vi "WILT Find And Reserve Semaphore.vi"(8 "error in (no error)":errorcluster, 10 "Semaphore":T1[](array[typedef]), 11 "VISA Refnum in":refnum<visa-resource-name>) -> (0 "error out":errorcluster, 2 "Skip Semaphore":bool, 3 "Refnum out":T1)   [LabVIEW 2016]
uses:
  <vilib>/Utility/error.llb/whitespace.ctl
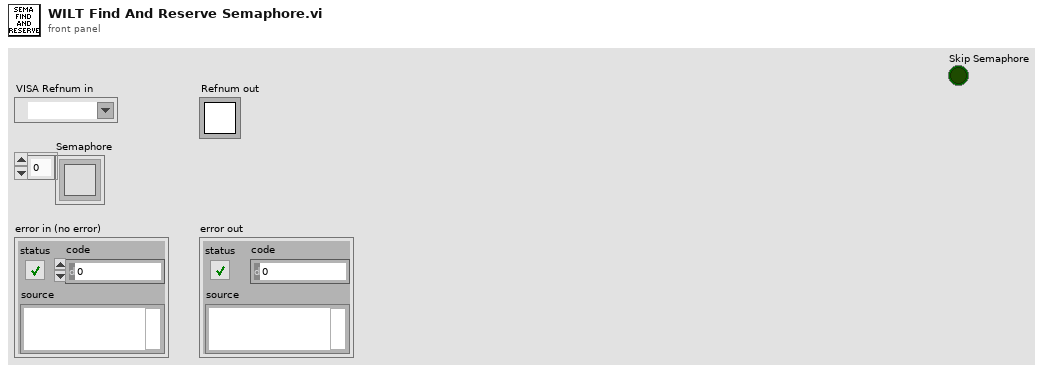
[diagram p1: front panel]
types:
  T1 = typedef "Semaphore RefNum" = refnum<k1>
  T2 = typedef "whitespace.ctl" = u16
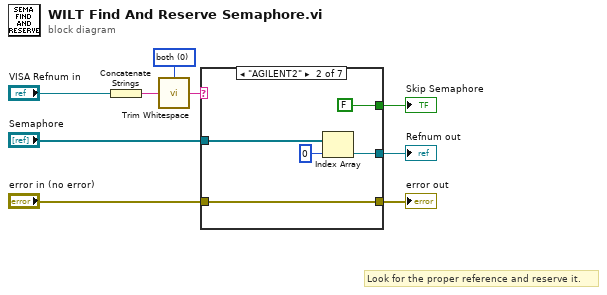
[diagram p0: block diagram]
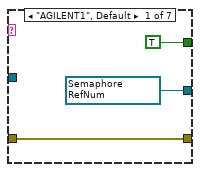
[diagram p2: hidden frame]
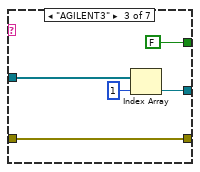
[diagram p3: hidden frame]
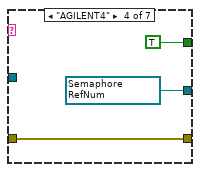
[diagram p4: hidden frame]
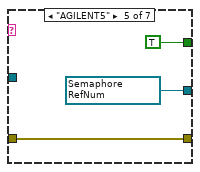
[diagram p5: hidden frame]
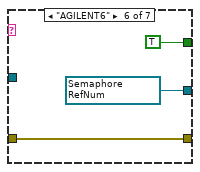
[diagram p6: hidden frame]
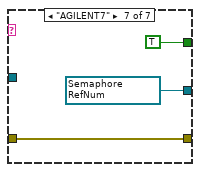
[diagram p7: hidden frame]
diagram:
  w5 = T2 0 items=["both", "start of string", "end of string"] ("location (both)")
  # "Look for the proper reference and reserve it."
  n1 = Concatenate Strings("VISA Refnum in") -> (w4:string)
  n2 = call <vilib>:"Trim Whitespace.vi"("string"=w4, "location (both)"=w5) -> ("trimmed string"=w6:string)
  n3 = case shown="\"AGILENT2\"" w6 {
    tunnel: "Semaphore" -> [_ w16 w21 _ _ _ _]
    tunnel: [w11 w15 w20 w24 w27 w30 w32] -> w7
    tunnel: [w12 w14 w19 w25 w28 w31 w34] -> w9
    tunnel: "error in (no error)" -> [w12 w14 w19 w25 w28 w31 w34]
    tunnel: [TRUE FALSE FALSE TRUE TRUE TRUE TRUE] -> w1
    frame "AGILENT1", Default {
      w11 = T1 refnum items=["semaphore"] ("Agilent")
    }
    frame "AGILENT2" {
      n4 = Index Array(array=w16, index=0) -> (element=w15:T1)
    }
    frame "AGILENT3" {
      n5 = Index Array(array=w21, index=1) -> (element=w20:T1)
    }
    frame "AGILENT4" {
      w24 = T1 refnum items=["semaphore"] ("Agilent")
    }
    frame "AGILENT5" {
      w27 = T1 refnum items=["semaphore"] ("Agilent")
    }
    frame "AGILENT6" {
      w30 = T1 refnum items=["semaphore"] ("Agilent")
    }
    frame "AGILENT7" {
      w32 = T1 refnum items=["semaphore"] ("Agilent")
    }
  }
  "error out" <- w9
  "Refnum out" <- w7
  "Skip Semaphore" <- w1
